vi "Run.vi"(6 "Type y_pred":T2(ring), 7 "Type y_true":T2(ring), 8 "error in (no error)":errorcluster caption="entrée d'erreur (pas d'erreur)", 9 "y_pred":string[][](array[string]), 10 "y_true":string[][](array[string]), 11 "Precision_RFS.lvclass":refnum<class "Precision_RFS.lvclass">) -> (0 "error out":errorcluster caption="sortie d'erreur", 2 "Data":T1, 3 "Precision_RFS.lvclass":refnum<class "Precision_RFS.lvclass">)   [LabVIEW 2020, in "Precision_RFS.lvclass"]
doc: "Returns :\n\n- precision : float (if average is not None) or array of float, shape = [n_unique_labels]\n- recall : float (if average is not None) or array of float, , shape = [n_unique_labels]\n- fbeta_score : float (if average is not None) or array of float, shape = [n_unique_labels]\n- support : None (if average is not None) or array of int, shape = [n_unique_labels]\nThe number of occurrences of each label in y_true."
uses:
  Precision_RFS.lvclass
  Precision_RFS.lvclass/Precision_RFS.ctl
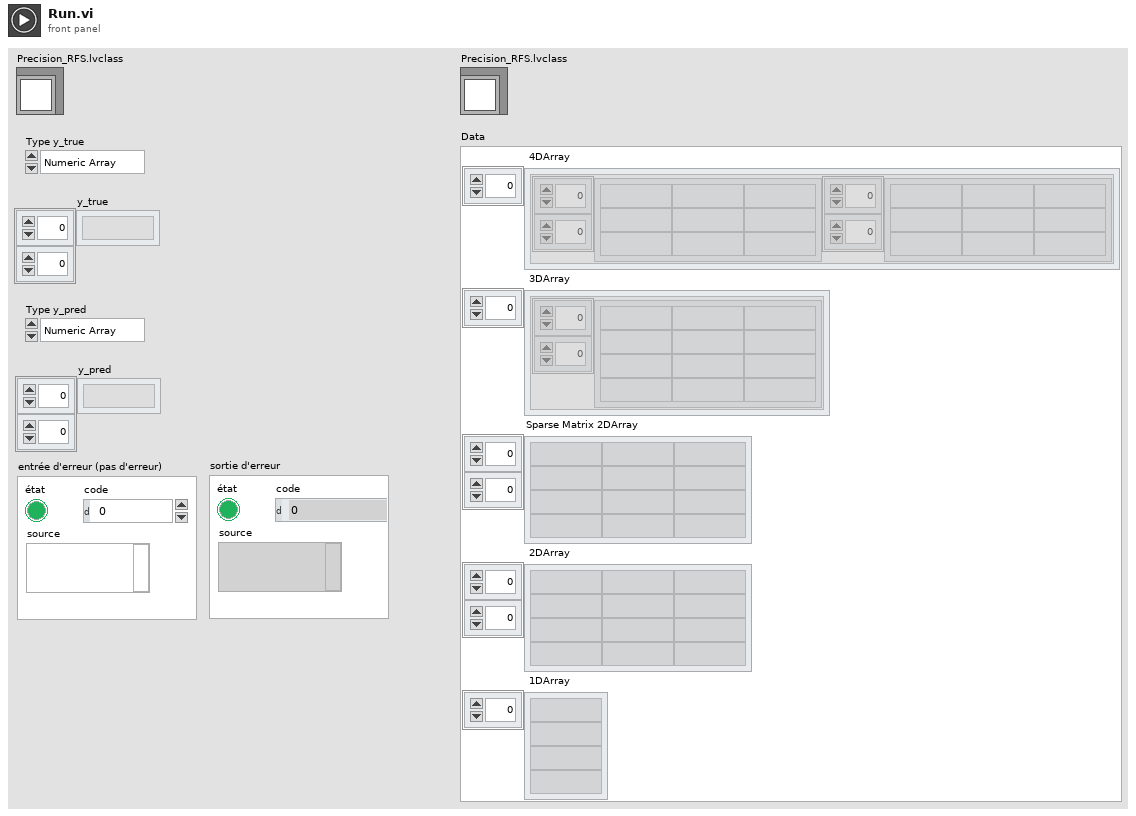
[diagram p1: front panel]
types:
  T1 = cluster{" 4DArray":cluster{"1":string[][], "2":string[][]}[], " 3DArray":cluster{"Tableau":string[][]}[], "Sparse Matrix 2DArray":string[][], " 2DArray":string[][], " 1DArray":string[]}
  T2 = enum16{"Numeric Array", "String Array", "Sparse"}
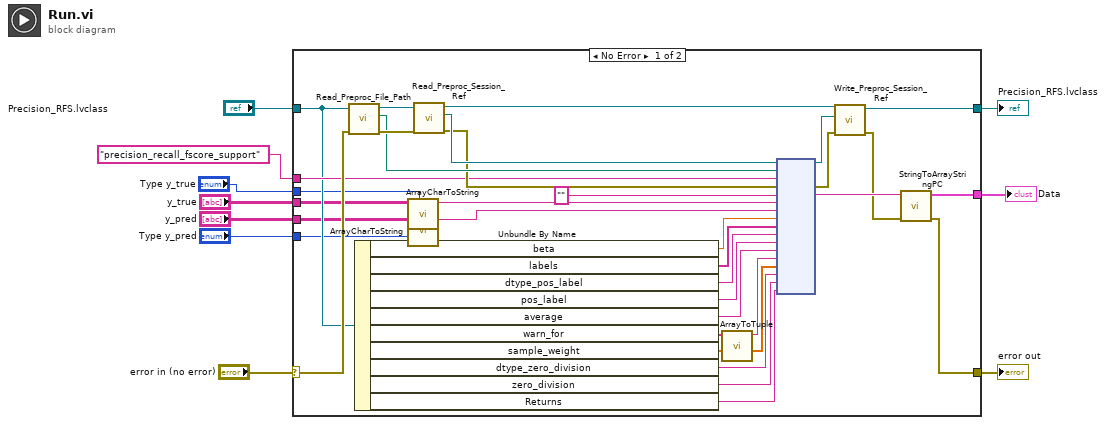
[diagram p0: block diagram]
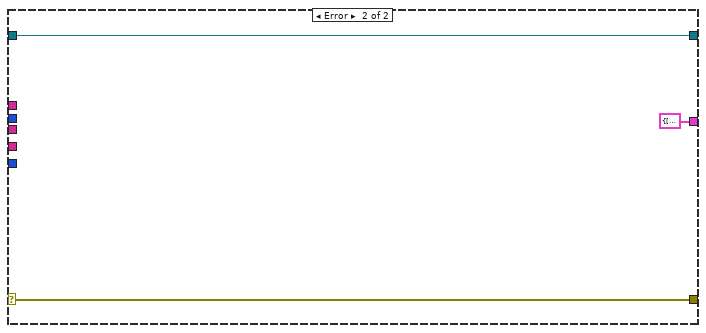
[diagram p2: hidden frame]
diagram:
  n1 = case shown="No Error" "error in (no error)" {
    selector: "error in (no error)" -> [w35 w47]
    tunnel: [w11 w47] -> w9
    tunnel: [w21 w46] -> w7
    tunnel: "Precision_RFS.lvclass" -> [w33 w46]
    tunnel: "precision_recall_fscore_support" -> [w34 _]
    tunnel: "y_true" -> [w20 _]
    tunnel: "y_pred" -> [w18 _]
    tunnel: "Type y_true" -> [w19 _]
    tunnel: "Type y_pred" -> [w17 _]
    tunnel: [w12 T1 {" 4DArray"=[], " 3DArray"=[], "Sparse Matrix 2DArray"=[], " 2DArray"=[], " 1DArray"=[]} ("Data")] -> w1
    frame No Error {
      n2 = call-dynamic "Read_Preproc_File_Path.vi"("error in (no error)"=w35, "Python in"=w33) -> ("error out"=w43:errorcluster, "File_Path"=w42:path, "Python out"=w44:refnum<class "Precision_RFS.lvclass">)  [unwired: 7 in]
      n3 = Unbundle By Name(w33) -> ("beta"=w32:dbl, "labels"=w31:string[], "dtype_pos_label"=w30:string, "pos_label"=w29:string, "average"=w28:string, "warn_for"=w27:string[], "sample_weight"=w25:dbl[], "dtype_zero_division"=w24:string, "zero_division"=w23:string, "Returns"=w22:string)
      n4 = call "ArrayCharToString.vi"("Type"=w19, "TAB"=w20) -> ("Instruction"=w16:string)  [unwired: 9 in]
      n5 = call "ArrayCharToString.vi"("Type"=w17, "TAB"=w18) -> ("Instruction"=w15:string)  [unwired: 9 in]
      n6 = call-dynamic "Read_Preproc_Session_Ref.vi"("error in (no error)"=w43, "Python in"=w44) -> ("error out"=w40:errorcluster, "Session_ref"=w41:refnum<k35>, "Python out"=w39:refnum<class "Precision_RFS.lvclass">)  [unwired: 7 in]
      n7 = call "ArrayToTuple.vi"("Tableau"=w27) -> ("Tuple"=w26:string)  [unwired: 10 in]
      n8 = node(w41, w42, w34, w40, "", w16, w15, w32, w31, w30, w29, w28, w26, w25, w24, w23, w22) -> (w37:refnum<k35>, w38:errorcluster, w14:string)  [unwired: 12 in, 2 out]
      n9 = call-dynamic "Write_Preproc_Session_Ref.vi"("error in (no error)"=w38, "Session_ref"=w37, "Python in"=w39) -> ("error out"=w13:errorcluster, "Python out"=w21:refnum<class "Precision_RFS.lvclass">)  [unwired: 7 in]
      n10 = call "StringToArrayStringPC.vi"("sortie d'erreur"=w13, "Return value"=w14) -> ("sortie d'erreur"=w11:errorcluster, "Data"=w12:T1)  [unwired: 8 in]
    }
    frame Error {
    }
  }
  "error out" <- w9
  "Precision_RFS.lvclass" <- w7
  "Data" <- w1
